vi "MovingDateTrans.vi"(2 "INPUT":dbl[](array[numeric])) -> (0 "MOVEING COMMAND":string)   [LabVIEW 2016]
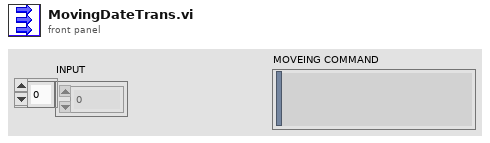
[diagram p1: front panel]
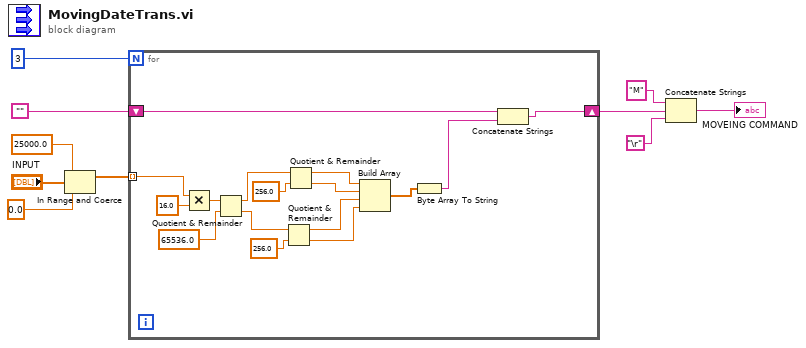
[diagram p0: block diagram]
diagram:
  n1 = In Range and Coerce ("判定范围并强制转换")(upper limit=25000.0 ("上限"), x="INPUT", lower limit=0.0 ("下限")) -> (coerced(x)=w3:dbl[])  [unwired: 1 out]
  n2 = for {
    N: 3 -> [_]
    tunnel: w3 -> [w21] mode=indexing
    shift-right: [w19] -> w8
    shift-left: "" -> [w20]
    n3 = Multiply(x=w21, y=16.0) -> (x*y=w23:dbl)
    n4 = Quotient & Remainder(x=w23, y=65536.0) -> (x-y*floor(x/y)=w25:dbl, floor(x/y)=w17:dbl)
    n5 = Quotient & Remainder(x=w17, y=256.0) -> (x-y*floor(x/y)=w14:dbl, floor(x/y)=w13:dbl)
    n6 = Quotient & Remainder(x=w25, y=256.0) -> (x-y*floor(x/y)=w16:dbl, floor(x/y)=w15:dbl)
    n7 = Build Array(w16, w15, w14, w13) -> (w12:dbl[])
    n8 = Byte Array To String(unsigned byte array=w12) -> (string=w11:string)
    n9 = Concatenate Strings(w20, w11) -> (w19:string)
  }
  n10 = Concatenate Strings("M" ("string"), w8, "\r") -> (→"MOVEING COMMAND":string)
